vi "params.From JSON Tree.vi"(8 "error in (no error)":errorcluster, 10 "JSON in":refnum<class "JSON Null.lvclass">, 11 "params in":refnum<class "params.lvclass">) -> (0 "error out":errorcluster, 3 "params in":refnum<class "params.lvclass">)   [LabVIEW 2016, in "params.lvclass"]
uses:
  params.lvclass
  <vilib>/NI/JSON Support for LabVIEW/JSON Data Classes/JSON Datatype/JSON Null.lvclass
  params.lvclass/params.ctl
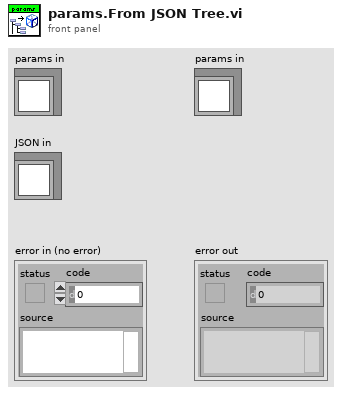
[diagram p1: front panel]
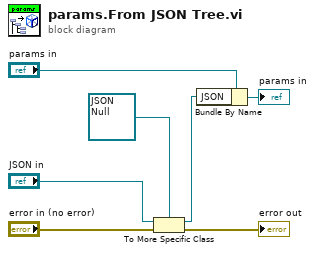
[diagram p0: block diagram]
diagram:
  n1 = To More Specific Class(target class=refnum<class "JSON Null.lvclass"> refnum ("JSON in"), reference="JSON in", error in="error in (no error)") -> (specific class reference=w4:refnum<class "JSON Null.lvclass">, error out=→"error out":errorcluster)
  n2 = Bundle By Name(cluster="params in", "JSON"=w4) -> (→"params in":refnum<class "params.lvclass">)
